vi "SV Test for Measurement Settled.vi"   [LabVIEW 2017]
doc: "Use this VI to test a settled double-precision output of an input array or waveform. Use the <B>settling configuration</B> input to configure the settling mask parameters. <B>output values</B> returns the thresholds and failures from the settling mask. Use the waveform instance of this VI to test waveform input."
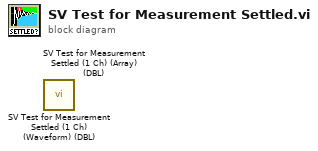
[diagram p0: block diagram]
diagram:
  n1 = call <vilib>:"SV Test for Measurement Settled (1 Ch) (Waveform) (DBL).vi"() -> ()  [unwired: 8 in, 4 out]
  n2 = call <vilib>:"SV Test for Measurement Settled (1 Ch) (Array) (DBL).vi"() -> ()  [unwired: 8 in, 4 out]
